vi "XML getApiCommands.vi"(10 "Commands In":T1[](array[typedef]), 11 "Commands XML":string) -> (2 "Commands Out":T1[](array[typedef]))   [LabVIEW 2011]
uses:
  Controls/PIM.API.Command.Unique.ctl
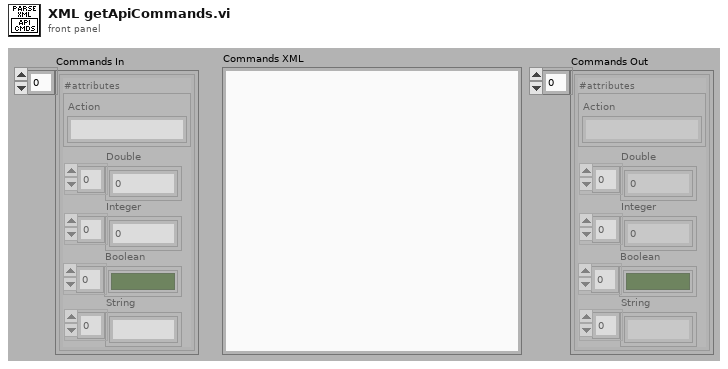
[diagram p1: front panel]
types:
  T1 = typedef "PIM.API.Command.Unique.ctl" = cluster{"#attributes":cluster{"Action":string}, "Double":dbl[], "Integer":i32[], "Boolean":bool[], "String":string[]}
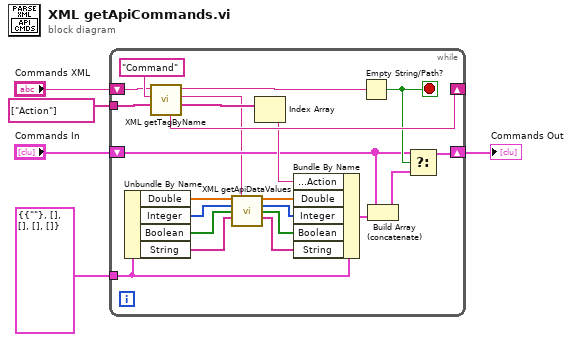
[diagram p0: block diagram]
diagram:
  n1 = while {
    shift-right: [w25] -> _
    shift-left: "Commands XML" -> [w26]
    shift-right: [w21] -> w5
    shift-left: "Commands In" -> [w18]
    tunnel: T1 {"#attributes"={"Action"=""}, "Double"=[], "Integer"=[], "Boolean"=[], "String"=[]} -> [w15]
    tunnel: string[] ["Action"] -> [w19]
    stop <- w20 stop-if-true
    n2 = Unbundle By Name(w15) -> ("Double"=w13:dbl[], "Integer"=w12:i32[], "Boolean"=w11:bool[], "String"=w10:string[])
    n3 = call "XML getTagByName.vi"("Get Attributes"=w19, "Tag Name"="Command", "XML String"=w26) -> ("Attribute Values"=w22:string[], "Tag Contents"=w14:string, "Matching Tag"=w24:string, "After Tag"=w25:string)  [unwired: 4 in, 1 out]
    n4 = call "XML getApiDataValues.vi"("Double in"=w13, "XML Data"=w14, "Integer in"=w12, "Boolean in"=w11, "String in"=w10) -> ("Double out"=w9:dbl[], "Integer out"=w8:i32[], "Boolean out"=w7:bool[], "String out"=w6:string[])  [unwired: 6 in, 1 out]
    n5 = Index Array(array=w22) -> (element=w23:string)  [unwired: 1 in]
    n6 = Bundle By Name(cluster=w15, "#attributes.Action"=w23, "Double"=w9, "Integer"=w8, "Boolean"=w7, "String"=w6) -> (w17:T1)
    n7 = Empty String/Path?(string/path=w24) -> (empty?=w20:bool)
    n8 = Build Array (concatenate)(w18, w17) -> (w16:T1[])
    n9 = Select(t=w18, s=w20, f=w16) -> (s? t:f=w21:T1[])
  }
  "Commands Out" <- w5
